vi "GetPathOfGitLog.vi"(11 "Path":path) -> (0 "git hash (version)":string, 1 "Branch":string, 2 "git log file path":path, 3 "git hash file path":path)   [LabVIEW 2018, in "feGEM DataPacker.lvlib"]
uses:
  feGEM DataPacker.lvlib
  <userlib>/_RADE/MTA-lib/file/file.llb/Build Path - Traditional__ogtk.vi
panel:
  out "Stripped ref path":string
  out "HEAD file substring":string
  out "HEAD file":string
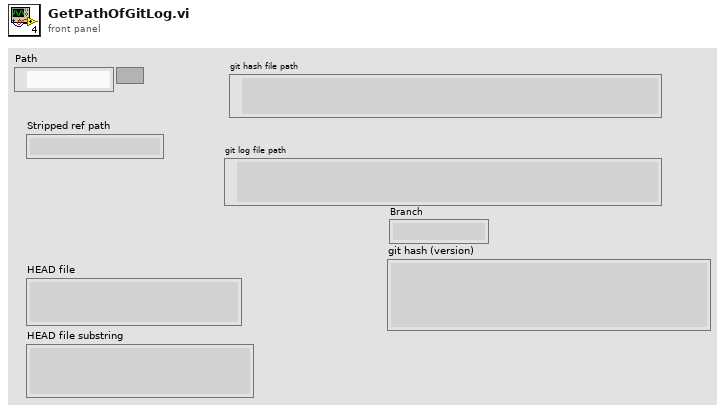
[diagram p1: front panel]
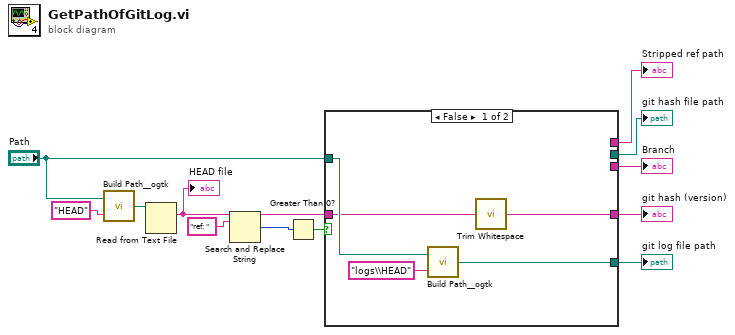
[diagram p0: block diagram]
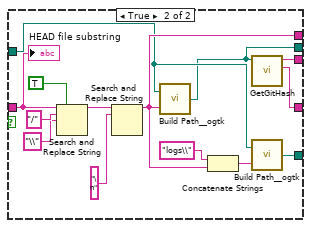
[diagram p2: hidden frame]
diagram:
  n1 = call-poly <userlib>:"Build Path__ogtk.vi"("name or relative path"="HEAD", "base path"="Path") -> ("appended path"=w12:path)
  n2 = Read from Text File(file (use dialog)=w12) -> (text=w11:string)  [unwired: 3 in, 3 out]
  "HEAD file" <- w11
  n3 = Search and Replace String(input string=w11, search string="ref: ") -> (result string=w7:string, number of replacements=w9:i32)  [unwired: 6 in, 2 out]
  n4 = Greater Than 0?(x=w9) -> (x > 0?=w8:bool)
  n5 = case shown="False" w8 {
    tunnel: "Path" -> [w18 w22]
    tunnel: w7 -> [w15 w25]
    tunnel: [_ w24] -> w5
    tunnel: [w17 w23] -> w4
    tunnel: [_ w21] -> w3
    tunnel: [_ w20] -> w2
    tunnel: [w14 w19] -> w1
    frame False {
      n6 = call-poly <userlib>:"Build Path__ogtk.vi"("name or relative path"="logs\\HEAD" ("replace string (\"\")"), "base path"=w18) -> ("appended path"=w17:path)
      n7 = call <vilib>:"Trim Whitespace.vi"("string"=w15) -> ("trimmed string"=w14:string)  [unwired: 1 in]
    }
    frame True {
      n8 = Search and Replace String(replace all?=TRUE ("replace all? (F)"), input string=w25, search string="/", replace string="\\" ("replace string (\"\")")) -> (result string=w32:string)  [unwired: 4 in, 3 out]
      n9 = Search and Replace String(input string=w32, search string="\n") -> (result string=w24:string)  [unwired: 6 in, 3 out]
      n10 = call-poly <userlib>:"Build Path__ogtk.vi"("name or relative path"=w24, "base path"=w22) -> ("appended path"=w21:path)
      n11 = Concatenate Strings("logs\\" ("replace string (\"\")"), w24) -> (w31:string)
      n12 = call "GetGitHash.vi"("git hash file path"=w21) -> ("git hash (version)"=w19:string, "Branch"=w20:string)  [unwired: 9 in]
      n13 = call-poly <userlib>:"Build Path__ogtk.vi"("name or relative path"=w31, "base path"=w22) -> ("appended path"=w23:path)
      "HEAD file substring" <- w25
    }
  }
  "Stripped ref path" <- w5
  "git log file path" <- w4
  "git hash file path" <- w3
  "Branch" <- w2
  "git hash (version)" <- w1
